vi "weizhiTEST-LAST.vi"() -> ()   [LabVIEW 2013]
panel:
  out "位置":dbl=10000.0
  in  "Change Velocity":dbl=1.0
  in  "Distance":dbl
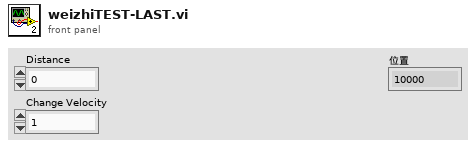
[diagram p1: front panel]
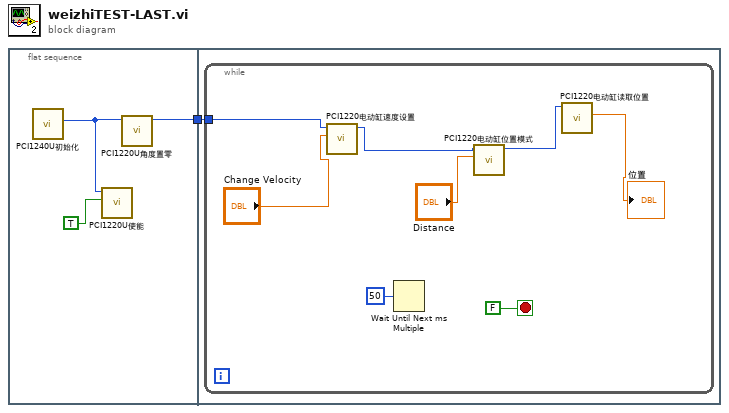
[diagram p0: block diagram]
diagram:
  n1 = flat-sequence {
    tunnel: [w4] -> w1
    tunnel: w1 -> [w5]
    frame #0 {
      n2 = call "PCI1240U初始化.vi"() -> ("1电机"=w2:u32)  [unwired: 6 in, 5 out]
      n3 = call "PCI1220U使能.vi"("使能"=TRUE, "AxisHandle IN"=w2) -> ()  [unwired: 9 in, 1 out]
      n4 = call "PCI1220U角度置零.vi"("AxisHandle IN"=w2) -> ("AxisHandle OUT"=w4:u32)  [unwired: 10 in]
    }
    frame #1 {
      n5 = while {
        tunnel: w5 -> [w9]
        stop <- FALSE stop-if-true
        n6 = call "PCI1220电动缸速度设置.vi"("Change Velocity"="Change Velocity", "AxisHandle IN"=w9) -> ("AxisHandle OUT"=w8:u32)  [unwired: 9 in]
        n7 = Wait Until Next ms Multiple(millisecond multiple=u32 50 ("毫秒倍数")) -> ()  [unwired: 1 out]
        n8 = call "PCI1220电动缸位置模式 .vi"("Distance"="Distance", "AxisHandle IN"=w8) -> ("AxisHandle OUT"=w7:u32)  [unwired: 8 in, 1 out]
        n9 = call "PCI1220电动缸读取位置.vi"("AxisHandle IN"=w7) -> ("位置"=→"位置":dbl)  [unwired: 9 in, 1 out]
      }
    }
  }
